vi "Find Target.vi"() -> ()   [LabVIEW 2014]
panel:
  out "Step Back":u32
  out "Scan Step Number":i32
  out "Scan Loop Number":i32
  out "IR_Range":dbl
  in  "stop":bool
  out "Sensor Scan":i16[][](graph)
  out "Real World":i32[][](graph)
  # "<-- USE THIS if the \nsub goes out of\ncontrol"
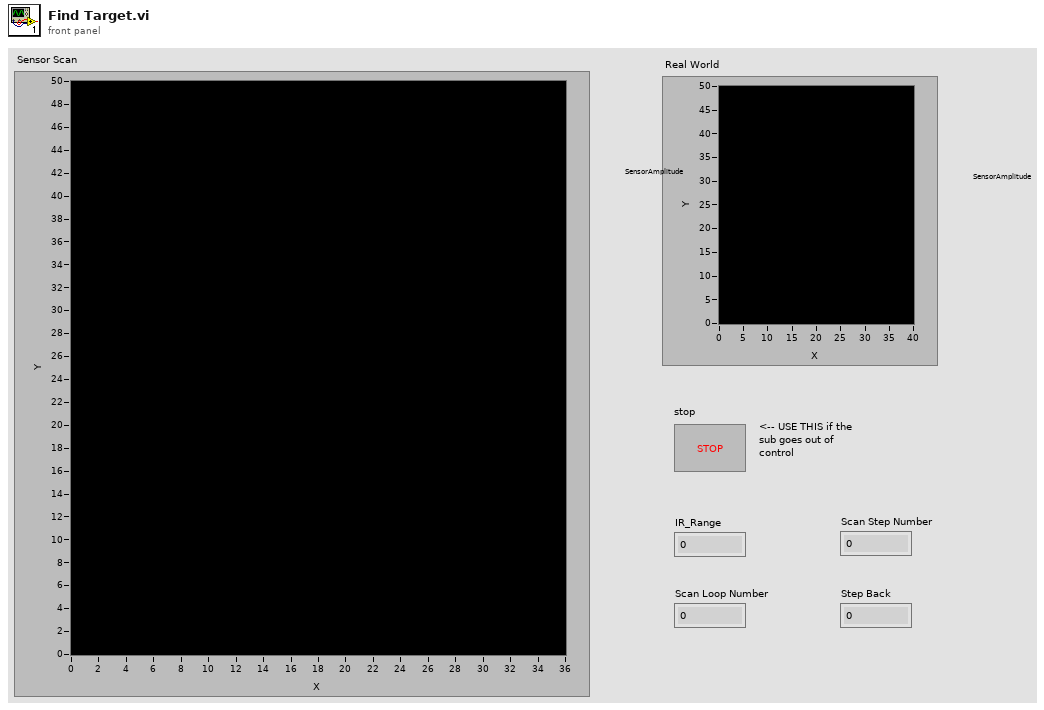
[diagram p1: front panel]
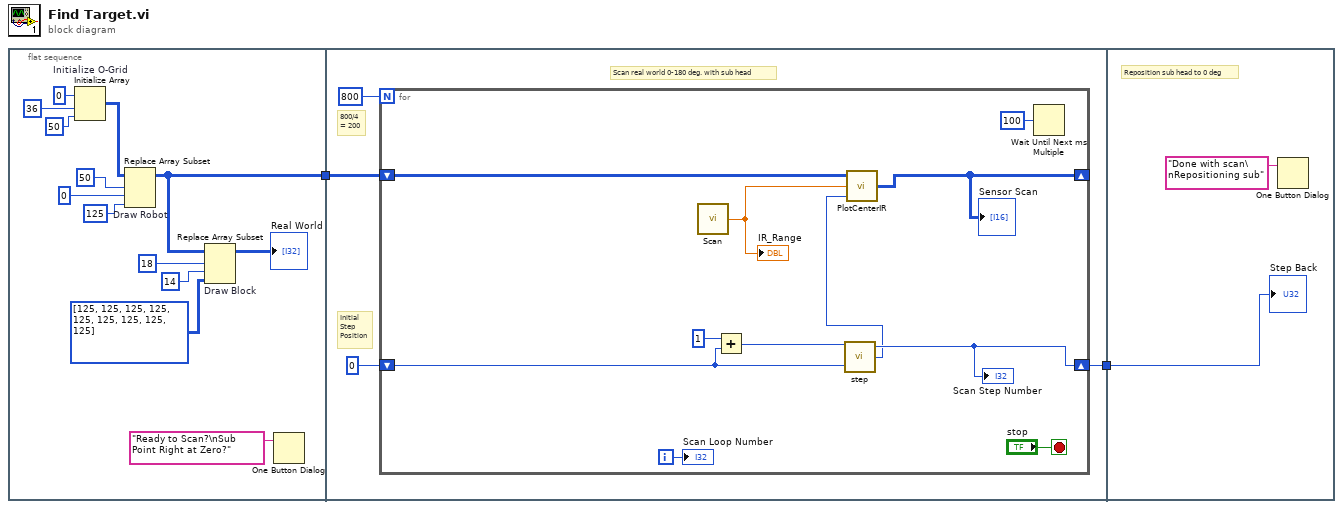
[diagram p0: block diagram]
diagram:
  n1 = flat-sequence {
    tunnel: [w3] -> w2
    tunnel: w2 -> [w18]
    tunnel: [w16] -> w1
    tunnel: w1 -> [w31]
    frame #0 {
      n2 = Initialize Array "Initialize O-Grid"(0 ("element"), 36 ("dimension size"), 50 ("dimension size")) -> (w11:i32[][])
      n3 = Replace Array Subset "Draw Robot"(array=w11, new element=125, index (row)=50, index (col)=0 ("element")) -> (w3:i32[][])
      n4 = Replace Array Subset "Draw Block"(array=w3, new element=i32[][] [[125, 125, 125], [125, 125, 125], [125, 125, 125]], index (row)=18, index (col)=14 ("disabled index (col)")) -> (→"Real World":i32[][])
      n5 = One Button Dialog(message="Ready to Scan?\nSub Point Right at Zero?") -> ()  [unwired: 1 in, 1 out]
    }
    frame #1 {
      # "Scan real world 0-180 deg. with sub head"
      # "800/4\n= 200"
      # "Initial\nStep\nPosition"
      n6 = for {
        N: 800 -> [_]
        shift-right: [w25] -> _
        shift-left: w18 -> [w26]
        shift-right: [w24] -> w16
        shift-left: 0 -> [w22]
        i -> [w30]
        stop <- "stop" stop-if-true
        n7 = call "Scan.vi"() -> ("IR_D_Center"=w20:dbl)  [unwired: 1 in]
        "IR_Range" <- w20
        n8 = Add(x=1, y=w22) -> (x+y=w23:i32)
        n9 = call "step.vi"("Desired Position"=w23, "Current Position"=w22) -> ("Position Out"=w24:i32, "Sensor Head Position"=w21:i32)  [unwired: 1 in]
        "Scan Step Number" <- w24
        n10 = call "PlotCenterIR.vi"("StepAngle"=w21, "IR_D"=w20, "InWorld"=w26) -> ("OutWorld"=w25:i16[][])
        "Sensor Scan" <- w25
        n11 = Wait Until Next ms Multiple(millisecond multiple=u32 100) -> ()  [unwired: 1 out]
        "Scan Loop Number" <- w30
      }
    }
    frame #2 {
      # "Reposition sub head to 0 deg"
      n12 = One Button Dialog(message="Done with scan\nRepositioning sub") -> ()  [unwired: 1 in, 1 out]
      "Step Back" <- w31
    }
  }
